vi "Write spectId.vi"(8 "error in (no error)":errorcluster, 10 "spectId":u16, 11 "StopImageCapture in":refnum<class "stopImageCapture.lvclass">) -> (0 "error out":errorcluster, 3 "StopImageCapture out":refnum<class "stopImageCapture.lvclass">)   [LabVIEW 2016, in "Commands.lvlib" / "stopImageCapture.lvclass"]
uses:
  stopImageCapture.lvclass
  stopImageCapture.lvclass/stopImageCapture.ctl
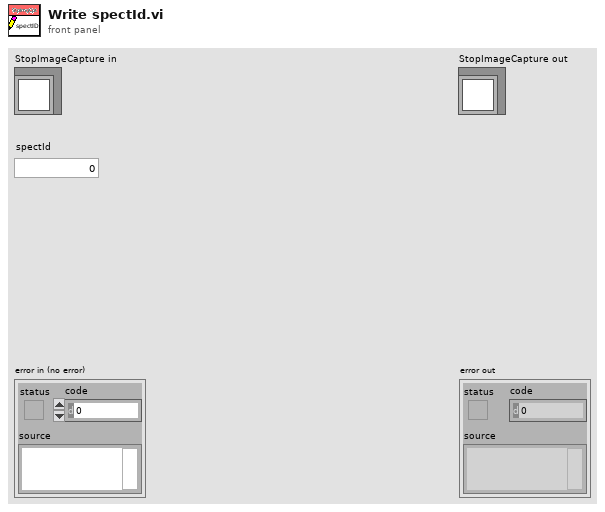
[diagram p1: front panel]
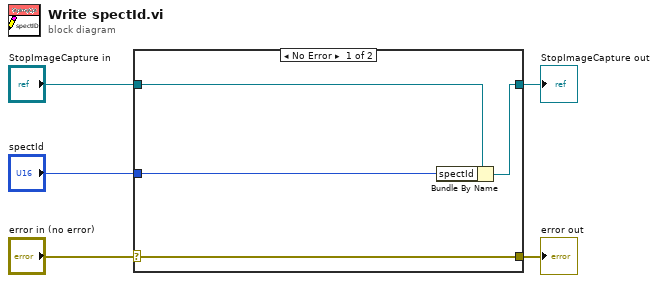
[diagram p0: block diagram]
diagram:
  n1 = case shown="No Error" "error in (no error)" {
    selector: "error in (no error)" -> [w9 w10]
    tunnel: [w9 w10] -> w4
    tunnel: [w7 w11] -> w2
    tunnel: "StopImageCapture in" -> [w8 w11]
    tunnel: "spectId" -> [w6 _]
    frame No Error {
      n2 = Bundle By Name(cluster=w8, "spectId"=w6) -> (w7:refnum<class "stopImageCapture.lvclass">)
    }
    frame Error {
    }
  }
  "error out" <- w4
  "StopImageCapture out" <- w2
